vi "FG Queue.vi"(7 "FG Actions":T1, 8 "error in (no error)":errorcluster, 11 "Message Queue":refnum<queue>) -> (0 "error out":errorcluster, 3 "Message Queue Out":refnum<queue>)   [LabVIEW 2020, in "COnfiguration Database.lvlib"]
doc: "This VI can Get, Set or release the queue reference used within the library it is part of."
uses:
  COnfiguration Database.lvlib
  Private Controls/Message Cluster.ctl
  Private Controls/Message enum.ctl
  Private Controls/FG Actions.ctl
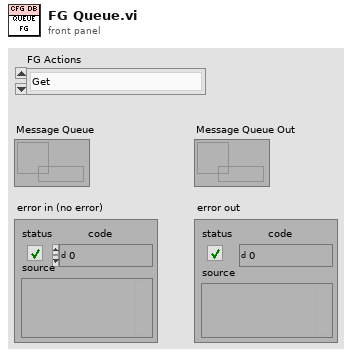
[diagram p1: front panel]
types:
  T1 = typedef "COnfiguration Database.lvlib/FG Actions.ctl" = enum16{"Get", "Set", "Clear"}
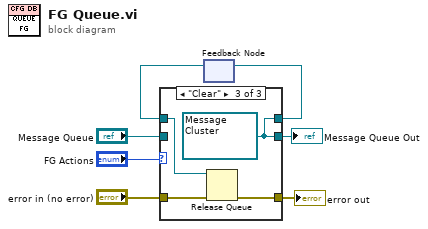
[diagram p0: block diagram]
diagram:
  n1 = feedback #1() -> (w3:refnum<queue>)  [unwired: 1 in]
  n2 = case shown="\"Clear\"" "FG Actions" {
    tunnel: "Message Queue" -> [_ w11 _]
    tunnel: [w8 w11 w14] -> w5
    tunnel: [w8 w11 w14] -> w4
    tunnel: w3 -> [w8 _ w15]
    tunnel: "error in (no error)" -> [w9 w10 w13]
    tunnel: [w9 w10 w12] -> w1
    frame "Get", Default {
    }
    frame "Set" {
    }
    frame "Clear" {
      w14 = refnum<queue> refnum ("Message Queue")
      n3 = Release Queue(queue=w15, error in (no error)=w13) -> (error out=w12:errorcluster)  [unwired: 1 in, 2 out]
    }
  }
  "Message Queue Out" <- w5
  "error out" <- w1
  n4 = feedback-in #1(w4) -> ()
